vi "Flush Data to Log File.vi"(8 "error in (no error)":T1 caption="entrée d'erreur (pas d'erreur)", 10 "File d'attente de données":refnum<queue>, 11 "Configuration de l'enregistrement":T2) -> (0 "error out":T1 caption="sortie d'erreur")   [LabVIEW 2018, in "Logging.lvlib"]
doc: "Retirer de la file d'attente toutes les données en attente et les écrire dans le fichier journal. Fermer la référence de fichier TDMS."
uses:
  Logging.lvlib
  Logging Configuration.ctl
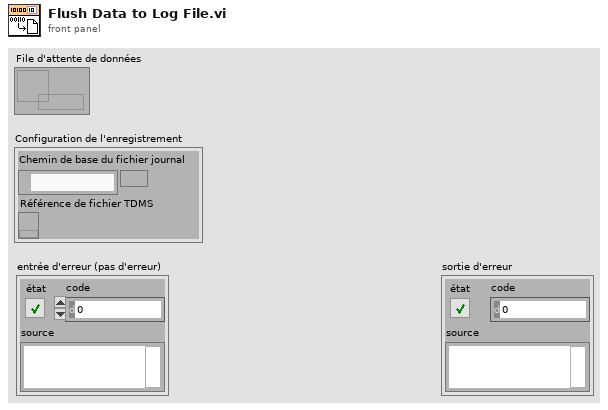
[diagram p1: front panel]
types:
  T1 = cluster{"état":bool, "code":i32, "source":string}
  T2 = typedef "Logging.lvlib/Logging Configuration.ctl" = cluster{"Chemin de base du fichier journal":path, "Référence de fichier TDMS":refnum<k34>}
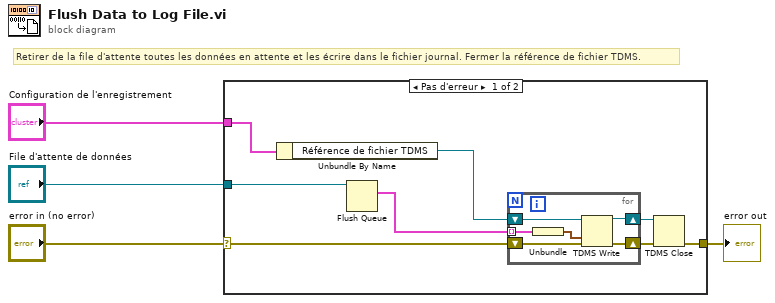
[diagram p0: block diagram]
diagram:
  # "Retirer de la file d'attente toutes les données en attente et les écrire dans le fichier journal. Fermer la référence de fichier TDMS."
  n1 = case shown="Pas d'erreur" "error in (no error)" {
    selector: "error in (no error)" -> [w5 w19]
    tunnel: "File d'attente de données" -> [w8 _]
    tunnel: "Configuration de l'enregistrement" -> [w7 _]
    tunnel: [w6 w19] -> w2
    frame No Error {
      n2 = Unbundle By Name(w7) -> ("Référence de fichier TDMS"=w9:refnum<k34>)
      n3 = Flush Queue(queue=w8) -> (remaining elements=w12:cluster{"Array":waveform(dbl)[]}[])  [unwired: 1 in, 2 out]
      n4 = for {
        shift-right: [w15] -> w10
        shift-left: w9 -> [w16]
        shift-right: [w17] -> w11
        shift-left: w5 -> [w18]
        tunnel: w12 -> [w14] mode=indexing
        n5 = Unbundle(w14) -> ("Array"=w13:waveform(dbl)[])
        n6 = TDMS Write(0:w16, 9:w13, 11:w18) -> (4:w15:refnum<k34>, 15:w17:errorcluster)  [unwired: 3 in, 2 out]
      }
      n7 = TDMS Close(8:w11, 11:w10) -> (0:w6:errorcluster)  [unwired: 1 out]
    }
    frame Error {
    }
  }
  "error out" <- w2
